vi "SpectralMeasurement_XMutation.vi"(0 "Diagram":refnum<vi>, 5 "ObjRef":refnum<vi>, 6 "Kind":string="SubVI", 7 "Information":string="<Not A Path>") -> (3 "Replace?":bool=TRUE)   [LabVIEW 2020]
uses:
  <vilib>/XNodeSupport/XNodeVersion.ctl
  <vilib>/XNodeSupport/NI_XNodeSupport.lvlib
  <vilib>/XNodeSupport/XNodeState.ctl
  <vilib>/XNodeSupport/XNodeUShort.ctl
  <vilib>/Utility/traverseref.llb/TRef TravTarget.ctl
  <vilib>/XNodeSupport/XNodeVariant.ctl
  <vilib>/Utility/miscctls.llb/LVPositionTypeDef.ctl
  <vilib>/express/express analysis/Spectral/XNode/ExpressSpectralMeasurementsBlockNode.xnode
  <vilib>/BlockNodeSupport/TerminalData.ctl
  <vilib>/picture/picture.llb/imagedata.ctl
  <vilib>/BlockNodeSupport/BlockNodeState.ctl
  <vilib>/XNodeSupport/XNodeType.ctl
  <vilib>/express/express shared/XNodes/controls/ExpressTerminalInfo.ctl
  <vilib>/express/express shared/XNodes/controls/ExpressState.ctl
  <vilib>/express/express shared/XNodes/controls/ExpressBlockNodeState.ctl
panel:
  in  "ExpressBlockNodeState":T1={"BlockNodeState"={"Terminal Data"=[{"Terminal Name"="Signals", "Terminal Display Name"="Signals", "Terminal ID"="Signals", "Terminal Flags"=517, "Terminal Type"=variant(waveform(dbl) {"t0"=timestamp(0 s since 1904-01-01), "dt"=0.0, "Y"=[]}), "Terminal Map ID"=0}, {"Terminal Name"="Selected Measurements", "Terminal Display Name"="Selected Measurements", "Terminal ID"="Selected Measurements", "Terminal Flags"=769, "Terminal Type"=variant(u32 0), "Terminal Map ID"=1}, {"Terminal Name"="Restart Averaging", "Terminal Display Name"="Restart Averaging", "Terminal ID"="Restart Averaging", "Terminal Flags"=769, "Terminal Type"=variant(bool FALSE), "Terminal Map ID"=2}, {"Terminal Name"="View", "Terminal Display Name"="View", "Terminal ID"="View", "Terminal Flags"=769, "Terminal Type"=variant(cluster{"dB On (F)":bool, "unwrap phase (F)":bool, "convert to degree (F)":bool} {"dB On (F)"=FALSE, "unwrap phase (F)"=FALSE, "convert to degree (F)"=FALSE}), "Terminal Map ID"=3}, {"Terminal Name"="Spectrum Window", "Terminal Display Name"="Spectrum Window", "Terminal ID"="Spectrum Window", "Terminal Flags"=769, "Terminal Type"=variant(u16 0), "Terminal Map ID"=4}, {"Terminal Name"="Spectrum Averaging Parameters", "Terminal Display Name"="Spectrum Averaging Parameters", "Terminal ID"="Spectrum Averaging Parameters", "Terminal Flags"=769, "Terminal Type"=variant(cluster{"averaging mode":u16, "weighting mode":u16, "number of averages":u32} {"averaging mode"=0, "weighting mode"=0, "number of averages"=0}), "Terminal Map ID"=5}, {"Terminal Name"="All Spectra", "Terminal Display Name"="All Spectra", "Terminal ID"="All Spectra", "Terminal Flags"=769, "Terminal Type"=variant(bool FALSE), "Terminal Map ID"=6}, {"Terminal Name"="error in (no error)", "Terminal Display Name"="error in (no error)", "Terminal ID"="error in (no error)", "Terminal Flags"=513, "Terminal Type"=variant(errorcluster {"status"=FALSE, "code"=0, "source"=""}), "Terminal Map ID"=7}, {"Terminal Name"="Measurement Output", "Terminal Display Name"="Measurement Output", "Terminal ID"="Measurement Output", "Terminal Flags"=525, "Terminal Type"=variant(dynamicdata []), "Terminal Map ID"=8}, {"Terminal Name"="averaging done", "Terminal Display Name"="averaging done", "Terminal ID"="averaging done", "Terminal Flags"=777, "Terminal Type"=variant(bool FALSE), "Terminal Map ID"=9}, {"Terminal Name"="Phase", "Terminal Display Name"="Phase", "Terminal ID"="Phase", "Terminal Flags"=777, "Terminal Type"=variant(dynamicdata []), "Terminal Map ID"=10}, {"Terminal Name"="error out", "Terminal Display Name"="error out", "Terminal ID"="error out", "Terminal Flags"=521, "Terminal Type"=variant(errorcluster {"status"=FALSE, "code"=0, "source"=""}), "Terminal Map ID"=11}], "Instance Name"="Spectral Measurements", "Type Name"="Spectral Measurements", "Draw Style"=1, "Connector Pane Pattern"=4833, "Flags"=370, "Grown Terminal List Order"=[], "Image"={"image type"=0, "image depth"=8, "image"=[0, 0, 255, 255, 255, 255, 255, 255, 255, 255, 255, 255, 255, 255, 255, 255, 255, 255, 255, 255, 255, 255, 255, 255, 255, 255, 255, 255, 255, 255, 0, 0, 0, 255, 210, 210, 210, 210, 210, 210, 210, 210, 210, 210, 210, 210, 210, 210, 210, 210, 210, 210, 210, 210, 210, 210, 210, 210, 210, 210, 210, 210, 255, 0, 255, 210, 210, 210, 210, 210, 210, 210, 210, 210, 210, 210, 210, 210, 210, 210, 210, 210, 210, 210, 210, 210, 210, 210, 210, 210, 210, 210, 210, 210, 210, 255, 255, 0, 0, 0, 0, 0, 0, 0, 0, 0, 0, 0, 0, 0, 0, 0, 0, 0, 0, 0, 0, 0, 0, 0, 0, 0, 0, 0, 0, 0, 0, 255, 255, 0, 0, 0, 0, 0, 0, 0, 0, 0, 0, 0, 0, 0, 0, 0, 0, 0, 0, 0, 0, 0, 0, 0, 0, 0, 0, 0, 0, 0, 0, 255, 255, 0, 0, 0, 0, 0, 0, 0, 0, 0, 0, 0, 0, 0, 0, 86, 86, 86, 86, 86, 86, 86, 86, 86, 86, 86, 86, 86, 86, 86, 86, 255, 255, 0, 0, 0, 0, 0, 0, 0, 0, 0, 0, 0, 0, 0, 0, 255, 255, 255, 255, 255, 255, 255, 255, 255, 255, 255, 255, 255, 255, 255, 255, 255, 255, 0, 0, 250, 250, 0, 0, 0, 0, 0, 0, 0, 0, 0, 0, 255, 5, 5, 5, 5, 5, 5, 5, 5, 5, 5, 5, 5, 5, 5, 5, 255, 255, 0, 0, 0, 250, 0, 0, 0, 0, 0, 0, 0, 0, 0, 0, 255, 5, 255, 5, 5, 5, 255, 5, 5, 5, 255, 5, 5, 5, 255, 5, 255, 255, 0, 0, 0, 250, 0, 0, 0, 0, 0, 0, 0, 0, 0, 0, 255, 5, 255, 5, 255, 5, 255, 5, 255, 5, 255, 5, 255, 5, 255, 5, 255, 255, 0, 0, 0, 250, 0, 0, 0, 0, 0, 0, 0, 0, 0, 0, 255, 255, 255, 255, 255, 255, 255, 255, 255, 255, 255, 255, 255, 255, 255, 255, 255, 255, 0, 0, 250, 250, 0, 0, 0, 0, 0, 0, 0, 0, 0, 0, 0, 0, 0, 0, 0, 0, 0, 0, 0, 0, 0, 0, 0, 0, 0, 0, 255, 255, 0, 0, 0, 250, 0, 0, 0, 0, 0, 0, 0, 0, 0, 0, 0, 0, 0, 0, 0, 0, 0, 0, 0, 0, 0, 0, 0, 0, 0, 0, 255, 255, 0, 0, 0, 250, 0, 0, 0, 0, 0, 0, 0, 0, 0, 0, 0, 0, 0, 0, 0, 0, 0, 0, 0, 0, 0, 0, 0, 0, 0, 0, 255, 255, 0, 0, 0, 250, 0, 0, 0, 0, 255, 0, 0, 0, 0, 0, 0, 0, 0, 0, 0, 0, 0, 0, 0, 0, 0, 0, 0, 0, 0, 0, 255, 255, 0, 0, 250, 250, 0, 0, 0, 0, 255, 0, 0, 0, 0, 0, 0, 0, 0, 0, 0, 0, 0, 0, 0, 0, 0, 0, 0, 0, 0, 0, 255, 255, 0, 0, 0, 250, 0, 0, 0, 0, 255, 0, 0, 0, 0, 0, 0, 0, 0, 0, 0, 0, 0, 0, 0, 0, 0, 0, 0, 0, 0, 0, 255, 255, 0, 0, 0, 250, 0, 0, 0, 0, 255, 0, 0, 0, 0, 0, 0, 0, 0, 0, 0, 0, 0, 0, 0, 0, 0, 0, 0, 0, 0, 0, 255, 255, 0, 0, 0, 250, 0, 0, 0, 0, 255, 0, 0, 0, 0, 0, 0, 0, 0, 0, 0, 0, 0, 0, 0, 0, 0, 0, 0, 0, 0, 0, 255, 255, 0, 0, 250, 250, 0, 0, 0, 0, 255, 0, 0, 0, 0, 0, 0, 0, 0, 0, 0, 0, 0, 0, 0, 0, 0, 0, 0, 0, 0, 0, 255, 255, 0, 0, 0, 250, 0, 0, 0, 255, 255, 255, 0, 0, 0, 0, 0, 0, 0, 0, 0, 0, 0, 0, 0, 0, 0, 0, 0, 0, 0, 0, 255, 255, 0, 0, 0, 250, 0, 0, 0, 255, 255, 255, 0, 0, 0, 0, 0, 0, 0, 0, 0, 0, 0, 0, 0, 0, 0, 0, 0, 0, 0, 0, 255, 255, 0, 0, 0, 250, 0, 0, 0, 255, 255, 255, 255, 0, 0, 0, 0, 0, 0, 0, 0, 0, 0, 0, 0, 0, 0, 0, 0, 0, 0, 0, 255, 255, 0, 0, 250, 250, 0, 0, 255, 255, 0, 0, 255, 0, 0, 0, 0, 0, 0, 0, 0, 0, 0, 0, 0, 0, 0, 0, 0, 0, 0, 0, 255, 255, 0, 0, 0, 250, 255, 255, 255, 255, 0, 0, 255, 255, 0, 0, 0, 0, 0, 0, 0, 0, 0, 0, 0, 0, 0, 0, 0, 0, 0, 0, 255, 255, 0, 0, 0, 250, 0, 255, 0, 0, 0, 0, 0, 255, 255, 255, 255, 255, 255, 255, 255, 255, 255, 255, 255, 255, 255, 255, 0, 0, 0, 0, 255, 255, 0, 0, 0, 250, 0, 0, 0, 0, 0, 0, 0, 0, 0, 0, 0, 0, 0, 0, 0, 0, 0, 0, 0, 0, 0, 0, 0, 0, 0, 0, 255, 255, 0, 0, 250, 250, 250, 250, 250, 250, 250, 250, 250, 250, 250, 250, 250, 250, 250, 250, 250, 250, 250, 250, 250, 250, 250, 250, 250, 250, 0, 0, 255, 255, 0, 0, 0, 250, 0, 0, 0, 250, 0, 0, 0, 250, 0, 0, 0, 250, 0, 0, 0, 250, 0, 0, 0, 250, 0, 0, 0, 250, 0, 0, 255, 255, 0, 0, 0, 0, 0, 0, 0, 0, 0, 0, 0, 0, 0, 0, 0, 0, 0, 0, 0, 0, 0, 0, 0, 0, 0, 0, 0, 0, 0, 0, 255, 0, 255, 0, 0, 0, 0, 0, 0, 0, 0, 0, 0, 0, 0, 0, 0, 0, 0, 0, 0, 0, 0, 0, 0, 0, 0, 0, 0, 0, 0, 255, 0, 0, 0, 255, 255, 255, 255, 255, 255, 255, 255, 255, 255, 255, 255, 255, 255, 255, 255, 255, 255, 255, 255, 255, 255, 255, 255, 255, 255, 255, 255, 0, 0], "mask"=[63, 255, 255, 252, 127, 255, 255, 254, 255, 255, 255, 255, 255, 255, 255, 255, 255, 255, 255, 255, 255, 255, 255, 255, 255, 255, 255, 255, 255, 255, 255, 255, 255, 255, 255, 255, 255, 255, 255, 255, 255, 255, 255, 255, 255, 255, 255, 255, 255, 255, 255, 255, 255, 255, 255, 255, 255, 255, 255, 255, 255, 255, 255, 255, 255, 255, 255, 255, 255, 255, 255, 255, 255, 255, 255, 255, 255, 255, 255, 255, 255, 255, 255, 255, 255, 255, 255, 255, 255, 255, 255, 255, 255, 255, 255, 255, 255, 255, 255, 255, 255, 255, 255, 255, 255, 255, 255, 255, 255, 255, 255, 255, 255, 255, 255, 255, 255, 255, 255, 255, 127, 255, 255, 254, 63, 255, 255, 252], "colors"=[16777215, 16777164, 16777113, 16777062, 16777011, 16776960, 16764159, 16764108, 16764057, 16764006, 16763955, 16763904, 16751103, 16751052, 16751001, 16750950, 16750899, 16750848, 16738047, 16737996, 16737945, 16737894, 16737843, 16737792, 16724991, 16724940, 16724889, 16724838, 16724787, 16724736, 16711935, 16711884, 16711833, 16711782, 16711731, 16711680, 13434879, 13434828, 13434777, 13434726, 13434675, 13434624, 13421823, 13421772, 13421721, 13421670, 13421619, 13421568, 13408767, 13408716, 13408665, 13408614, 13408563, 13408512, 13395711, 13395660, 13395609, 13395558, 13395507, 13395456, 13382655, 13382604, 13382553, 13382502, 13382451, 13382400, 13369599, 13369548, 13369497, 13369446, 13369395, 13369344, 10092543, 10092492, 10092441, 10092390, 10092339, 10092288, 10079487, 10079436, 10079385, 10079334, 10079283, 10079232, 10066431, 10066380, 10066329, 10066278, 10066227, 10066176, 10053375, 10053324, 10053273, 10053222, 10053171, 10053120, 10040319, 10040268, 10040217, 10040166, 10040115, 10040064, 10027263, 10027212, 10027161, 10027110, 10027059, 10027008, 6750207, 6750156, 6750105, 6750054, 6750003, 6749952, 6737151, 6737100, 6737049, 6736998, 6736947, 6736896, 6724095, 6724044, 6723993, 6723942, 6723891, 6723840, 6711039, 6710988, 6710937, 6710886, 6710835, 6710784, 6697983, 6697932, 6697881, 6697830, 6697779, 6697728, 6684927, 6684876, 6684825, 6684774, 6684723, 6684672, 3407871, 3407820, 3407769, 3407718, 3407667, 3407616, 3394815, 3394764, 3394713, 3394662, 3394611, 3394560, 3381759, 3381708, 3381657, 3381606, 3381555, 3381504, 3368703, 3368652, 3368601, 3368550, 3368499, 3368448, 3355647, 3355596, 3355545, 3355494, 3355443, 3355392, 3342591, 3342540, 3342489, 3342438, 3342387, 3342336, 65535, 65484, 65433, 65382, 65331, 65280, 52479, 52428, 52377, 52326, 52275, 52224, 39423, 39372, 39321, 39270, 39219, 39168, 26367, 26316, 26265, 26214, 26163, 26112, 13311, 13260, 13209, 13158, 13107, 13056, 255, 204, 153, 102, 51, 15597568, 14483456, 12255232, 11141120, 8912896, 7798784, 5570560, 4456448, 2228224, 1114112, 60928, 56576, 47872, 43520, 34816, 30464, 21760, 17408, 8704, 4352, 238, 221, 187, 170, 136, 119, 85, 68, 34, 17, 15658734, 14540253, 12303291, 11184810, 8947848, 7829367, 5592405, 4473924, 2236962, 1118481, 0], "Rectangle"={"left"=0, "top"=0, "right"=32, "bottom"=32}}}, "ExpressState"={"Terminal Info"=[{"types to adapt"=["ExpressData", "Waveform", "1D Array Waveform"], "show config value"=FALSE, "default type"=variant(waveform(dbl) {"t0"=timestamp(0 s since 1904-01-01), "dt"=0.0, "Y"=[]}), "display name control"=""}, {"types to adapt"=["Numeric"], "show config value"=FALSE, "default type"=variant(u32 0), "display name control"=""}, {"types to adapt"=["Boolean"], "show config value"=FALSE, "default type"=variant(bool FALSE), "display name control"=""}, {"types to adapt"=[""], "show config value"=FALSE, "default type"=variant(cluster{"dB On (F)":bool, "unwrap phase (F)":bool, "convert to degree (F)":bool} {"dB On (F)"=FALSE, "unwrap phase (F)"=FALSE, "convert to degree (F)"=FALSE}), "display name control"=""}, {"types to adapt"=["Numeric"], "show config value"=FALSE, "default type"=variant(u16 0), "display name control"=""}, {"types to adapt"=[""], "show config value"=FALSE, "default type"=variant(cluster{"averaging mode":u16, "weighting mode":u16, "number of averages":u32} {"averaging mode"=0, "weighting mode"=0, "number of averages"=0}), "display name control"=""}, {"types to adapt"=["Boolean"], "show config value"=FALSE, "default type"=variant(bool FALSE), "display name control"=""}, {"types to adapt"=[""], "show config value"=FALSE, "default type"=variant(errorcluster {"status"=FALSE, "code"=0, "source"=""}), "display name control"=""}, {"types to adapt"=["ExpressData"], "show config value"=FALSE, "default type"=variant(dynamicdata []), "display name control"="output name"}, {"types to adapt"=["Boolean"], "show config value"=FALSE, "default type"=variant(bool FALSE), "display name control"=""}, {"types to adapt"=["ExpressData"], "show config value"=FALSE, "default type"=variant(dynamicdata []), "display name control"=""}, {"types to adapt"=[""], "show config value"=FALSE, "default type"=variant(errorcluster {"status"=FALSE, "code"=0, "source"=""}), "display name control"=""}], "config control names"=[], "config data strings"=[], "config control data"=[variant(enum32{"Magnitude (RMS)", "Magnitude (Peak)", "Power spectrum", "Power spectral density"} enum."Magnitude (RMS)"), variant(enum32{"Linear", "dB"} enum."dB"), variant(u16 0), variant(bool FALSE), variant(enum32{"Vector", "RMS", "Peak hold"} enum."Vector"), variant(enum32{"Linear", "Exponential"} enum."Linear"), variant(u32 1), variant(enum32{"Every iteration", "Only when averaging complete"} enum."Every iteration"), variant(bool FALSE), variant(bool FALSE), variant(bool FALSE), variant(waveform(dbl)[] []), variant(waveform(dbl) {"t0"=timestamp(0 s since 1904-01-01), "dt"=1.0, "Y"=[]}), variant(errorcluster {"status"=FALSE, "code"=0, "source"=""}), variant(dynamicdata []), variant(cluster{"dB On (F)":bool, "unwrap phase (F)":bool, "convert to degree (F)":bool} {"dB On (F)"=FALSE, "unwrap phase (F)"=FALSE, "convert to degree (F)"=FALSE}), variant(cluster{"averaging mode":enum16{"No averaging", "Vector averaging", "RMS averaging", "Peak hold"}, "weighting mode":enum16{"Linear", "Exponential"}, "number of averages":u32} {"averaging mode"=enum."No averaging", "weighting mode"=enum."Linear", "number of averages"=0}), variant(string "Sample Data"), variant(string "Sample Result"), variant(waveform(dbl) {"t0"=timestamp(0 s since 1904-01-01), "dt"=1.0, "Y"=[]}), variant(string "Sample Result"), variant(string "Phase (rad.)"), variant(string "Phase (deg.)"), variant(bool FALSE), variant(bool FALSE), variant(string[] ["INsignal type", "INfrequency", "OUTsignal", "INphase", "INsamples per second"]), variant(string[] ["INsignal type", "INfrequency", "OUTsignal"]), variant(errorcluster {"status"=FALSE, "code"=0, "source"=""}), variant(bool FALSE), variant(dynamicdata []), variant(string[] ["FFT - (RMS)", "FFT - (Peak)", "Power Spectrum", "PSD"]), variant(string ""), variant(bool FALSE), variant(bool FALSE), variant(i32 0), variant(string ""), variant(bool FALSE), variant(bool FALSE), variant(bool FALSE), variant(enum16{"No averaging", "Vector averaging", "RMS averaging", "Peak hold"} enum."No averaging"), variant(enum16{"Linear", "Exponential"} enum."Linear"), variant(u32 0), variant(bool FALSE), variant(i32 0), variant(string "")], "units"=[], "configured?"=TRUE, "config VI path"=path "<vilib>/express/express analysis/Spectral/Config/ExnSpectralConfig Configure Spectral Measurements.vi", "block VI path"=path "<vilib>/express/express analysis/Spectral/Block/ExnSpectralBlock Spectral Measurements.vi", "config control labels"=["Selected Measurement", "Result", "Spectrum Window", "Averaging", "Mode", "Weighting", "Number of averages", "Produce Spectrum", "Unwrap phase", "Convert to degree", "Correction None", " Windowed Signal ", "Magnitude", "error out", "Signals", "View", "Spectrum Averaging Parameters", "Sample Input Signal", "Sample Magnitude Result", "Phase", "Sample Phase Result", "Phase (rad.)", "Phase (deg.)", "Restart Averaging", "okay out", "config terms", "config terms grown", "error in (no error)", "averaging done", "Measurement Output", "measurement names", "output name", "All Spectra", "status", "code", "source", "dB On (F)", "unwrap phase (F)", "convert to degree (F)", "averaging mode", "weighting mode", "number of averages", "status", "code", "source"], "show config value menu"=FALSE, "config value menu setting"=FALSE, "context help labels"=["Selected Measurement", "Result", "Spectrum Window", "Averaging", "Mode", "Weighting", "Number of averages", "Produce Spectrum", "Unwrap phase", "Convert to degree"], "valid help labels"=[]}} {"BlockNodeState"."Draw Style" items=["FunctionBlock", "ExpressVI", "Variable", "Elemental I/O", "32x32 Icon", "FunctionBlockCompact"]; "BlockNodeState"."Terminal Data"."Terminal Flags" format="%.0b"}
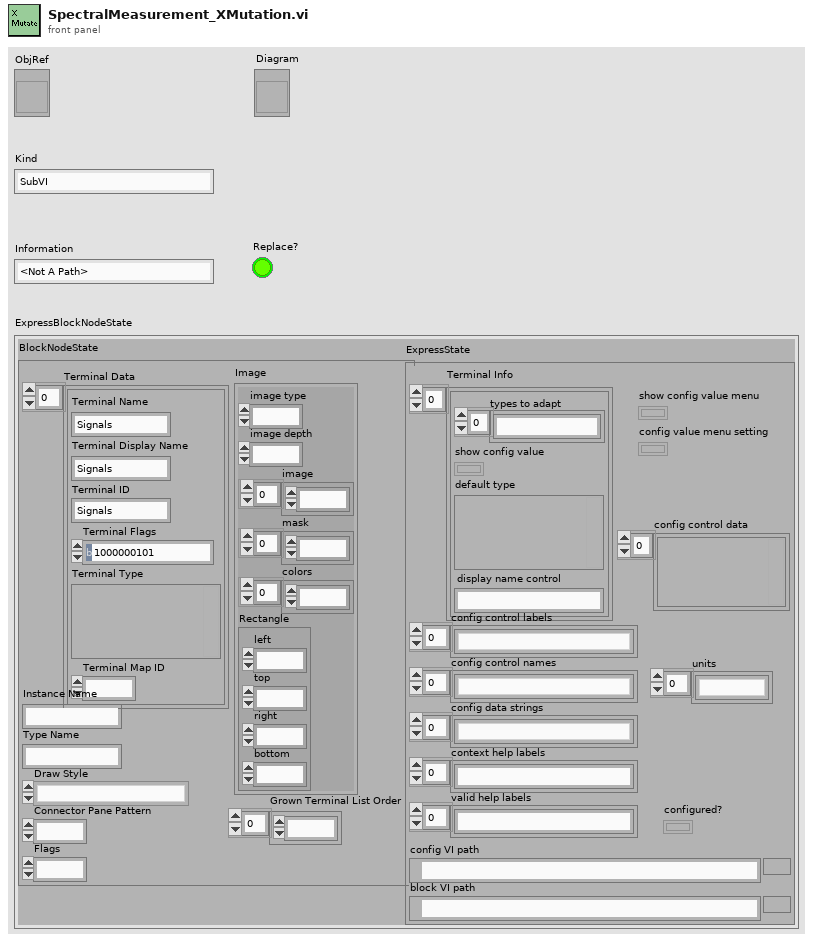
[diagram p1: front panel]
types:
  T1 = typedef "ExpressBlockNodeState.ctl" = cluster{"BlockNodeState":T2, "ExpressState":T5}
  T2 = typedef "BlockNodeState.ctl" = cluster{"Terminal Data":T3[], "Instance Name":string, "Type Name":string, "Draw Style":i32, "Connector Pane Pattern":i32, "Flags":i32, "Grown Terminal List Order":i32[], "Image":T4}
  T3 = typedef "TerminalData.ctl" = cluster{"Terminal Name":string, "Terminal Display Name":string, "Terminal ID":string, "Terminal Flags":i32, "Terminal Type":variant, "Terminal Map ID":i32}
  T4 = typedef "imagedata.ctl" = cluster{"image type":i32, "image depth":i32, "image":u8[], "mask":u8[], "colors":u32[], "Rectangle":cluster{"left":i16, "top":i16, "right":i16, "bottom":i16}}
  T5 = typedef "ExpressState.ctl" = cluster{"Terminal Info":T6, "config control names":string[], "config data strings":string[], "config control data":variant[], "units":string[], "configured?":bool, "config VI path":path, "block VI path":path, "config control labels":string[], "show config value menu":bool, "config value menu setting":bool, "context help labels":string[], "valid help labels":string[]}
  T6 = typedef "ExpressTerminalInfo.ctl" = cluster{"types to adapt":string[], "show config value":bool, "default type":T7, "display name control":string}[]
  T7 = typedef "NI_XNodeSupport.lvlib/XNodeType.ctl" = variant
  T8 = cluster{"dB On (F)":bool, "unwrap phase (F)":bool, "convert to degree (F)":bool}
  T9 = cluster{"averaging mode":enum16{"No averaging", "Vector averaging", "RMS averaging", "Peak hold"}, "weighting mode":enum16{"Linear", "Exponential"}, "number of averages":u32}
  T10 = typedef "TRef TravTarget.ctl" = enum16{"FP", "BD", "Other"}
  T11 = enum32{"Every iteration", "Only when averaging complete"}
  T12 = enum32{"Magnitude (RMS)", "Magnitude (Peak)", "Power spectrum", "Power spectral density"}
  T13 = typedef "NI_XNodeSupport.lvlib/XNodeState.ctl" = cluster{"Version":T14, "State Data":T16}
  T14 = typedef "NI_XNodeSupport.lvlib/XNodeVersion.ctl" = cluster{"Major":T15, "Minor":T15, "Fix":T15, "Build":T15}
  T15 = typedef "NI_XNodeSupport.lvlib/XNodeUShort.ctl" = u16
  T16 = typedef "NI_XNodeSupport.lvlib/XNodeVariant.ctl" = variant
  T17 = typedef "LVPositionTypeDef.ctl" = cluster{"Left":i32, "Top":i32}
  T18 = enum16{"No averaging", "Vector averaging", "RMS averaging", "Peak hold"}
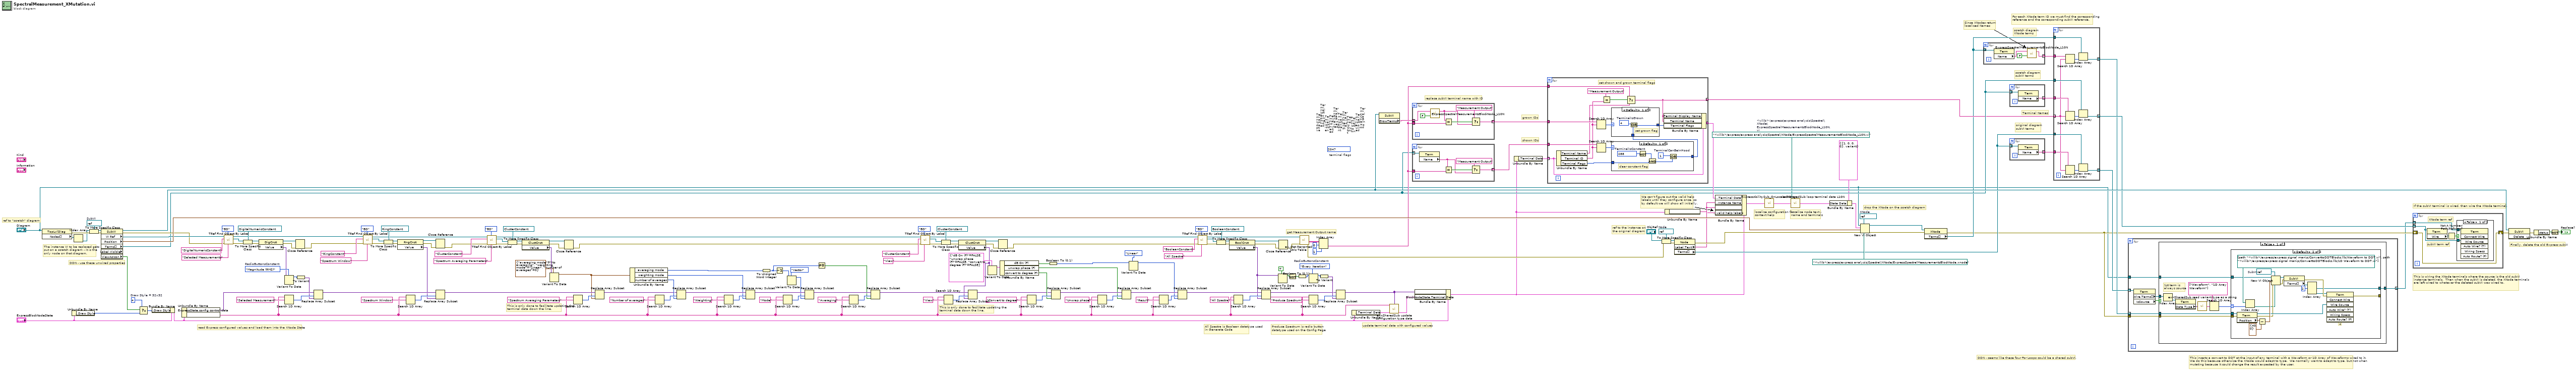
[diagram p0: block diagram]
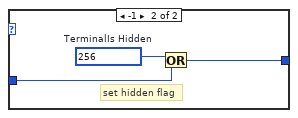
[diagram p4: hidden frame]
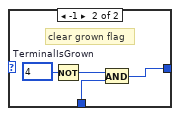
[diagram p5: hidden frame]
diagram:
  w3 = path "<vilib>/express/express analysis/Spectral/XNode/ExpressSpectralMeasurementsBlockNode_L10N.vi"  # <vilib>:\express\express analysis\Spectral\XNode\ExpressSpectralMeasurementsBlockNode_L10N.vi
  w21 = 4  # Draw Style = 32x32
  (unwired) 2047 ("TermFlags")
  w105 = T11."Every iteration"  # RadioButtonsConstant
  w65 = T12."Magnitude (RMS)"  # RadioButtonsConstant
  w184 = refnum<vi> refnum  # Node
  w191 = refnum<vi> refnum  # XNode
  w196 = refnum<vi> refnum  # SubVI
  # "Since XNodes return localized Names"
  # "We can't figure out the valid help labels until they configure once, so by default we will show all initially."
  # "localize node text - name and terminals"
  # "localize configuration for context help"
  # "scratch diagram\nXNode terms"
  # "scratch diagram\nsubVI terms"
  # "This inserts a convert to DDT at the input of any terminal with a Waveform or 1D Array of Waveforms wired to it.  We do this because otherwise the XNode would adapt to type.  We normally want to adapt to type, but not when mutating because it could change the result expected by the user."
  # "original diagram\nsubVI terms"
  # "Produce Spectrum is radio button datatype used on the Config Page"
  # "All Spectra is Boolean datatype used in Generate Code"
  # "DDN - seems like these four For Loops could be a shared subVI."
  # "DDN - use these unwired properties"
  # "This is only done to facilitate updating the terminal data down the line."
  # "TerminalIsAdaptive"
  # "TerminalIsRecommended"
  # "TerminalIsHidden"
  # "terminal flags"
  # "TerminalIsInverted"
  # "TerminalCanBeInverted"
  # "TerminalIsConstant"
  # "TerminalHilitedMask"
  # "TerminalIsOutput"
  # "TerminalIsGrown"
  # "TerminalIsRequired"
  # "TerminalCanBeInHood"
  # "This is only done to facilitate updating the terminal data down the line."
  # "update terminal data with configured values"
  # "Finally, delete the old Express subVI"
  # "For each XNode term ID we must find the corresponding reference and the corresponding subVI reference."
  # "drop the XNode on the scratch diagram"
  # "read Express configured values and load them into the XNode State"
  # "Terminal Names"
  # "If the subVI terminal is wired, then wire the XNode terminal."
  # "This is wiring the XNode terminals where the source is the old subVI instance terminals.  Then when the subVI is deleted, the XNode terminals are left wired to whatever the deleted subVI was wired to."
  # "The instance VI to be replaced gets put on a scratch diagram - it is the only node on that diagram."
  # "replace subVI terminal name with ID"
  # "grown IDs"
  # "shown IDs"
  # "get Measurement Output name"
  # "ref to \"scratch\" diagram"
  # "ref to the instance on the original diagram"
  n1 = property class="TopLvlDiag"(reference="Diagram") -> (error out=w195:errorcluster, "Nodes[]"=w197:refnum<vi>[])  [unwired: 1 in, 1 out]
  n2 = Unbundle By Name("ExpressBlockNodeState") -> ("BlockNodeState.Draw Style"=w20:i32)
  n3 = Index Array(array=w197) -> (element=w187:refnum<vi>)  [unwired: 1 in]
  n4 = To More Specific Class(target class=w196, reference=w187, error in=w195) -> (specific class reference=w193:refnum<vi>, error out=w194:errorcluster)
  n5 = property class="SubVI" props=["VI Ref", "Position", "Terms[]", "Label", "Visible", "ViewAsIcon"](reference=w193, error in=w194) -> (reference out=w91:refnum<vi>, error out=w172:errorcluster, "VI Ref"=w173:refnum<vi>, "Position"=w174:T17, "Terms[]"=w90:refnum<vi>[], "ViewAsIcon"=w22:bool)  [unwired: 1 out]
  n6 = Select(t=w21, s=w22, f=w20) -> (s? t:f=w23:i32)
  n7 = Bundle By Name(cluster="ExpressBlockNodeState", "BlockNodeState.Draw Style"=w23) -> (w24:T1)
  n8 = Unbundle By Name(w24) -> ("ExpressState.config control data"=w170:variant[], "ExpressState.config control labels"=w14:string[])
  n9 = call <vilib>:"TRef Find Object By Label.vi"("Label"="Selected Measurements", "Traverse Target"=TRef_TravTarget."BD", "error in (no error)"=w172, "Class Name"="DigitalNumericConstant" ("Label"), "VI Ref"=w173) -> ("error out"=w180:errorcluster, "Found Obj Ref"=w178:refnum<vi>, "dup VI Ref"=w157:refnum<vi>)  [unwired: 3 in, 1 out]
  n10 = To More Specific Class(target class=refnum<vi> refnum ("Other Refnum"), reference=w178, error in=w180) -> (specific class reference=w176:refnum<vi>, error out=w177:errorcluster)
  n11 = property class="DigCnst"(reference=w176, error in=w177) -> (reference out=w168:refnum<vi>, error out=w167:errorcluster, "Value"=w63:variant)
  n12 = Variant To Data(type=w65, Variant=w63) -> (data=w64:T12)  [unwired: 1 in, 1 out]
  n13 = Search 1D Array(1D array=w14, element="Selected Measurement" ("Label")) -> (index of element=w169:i32)  [unwired: 1 in]
  n14 = Close Reference(reference=w168, error in (no error)=w167) -> (error out=w156:errorcluster)
  n15 = To Variant(anything=w64) -> (Variant=w62:variant)
  n16 = Replace Array Subset(array=w170, new element=w62, index=w169) -> (w154:variant[])
  n17 = call <vilib>:"TRef Find Object By Label.vi"("Label"="Spectrum Window", "Traverse Target"=TRef_TravTarget."BD", "error in (no error)"=w156, "Class Name"="RingConstant" ("Label"), "VI Ref"=w157) -> ("error out"=w163:errorcluster, "Found Obj Ref"=w162:refnum<vi>, "dup VI Ref"=w141:refnum<vi>)  [unwired: 3 in, 1 out]
  n18 = To More Specific Class(target class=refnum<vi> refnum ("Other Refnum"), reference=w162, error in=w163) -> (specific class reference=w160:refnum<vi>, error out=w161:errorcluster)
  n19 = property class="RngCnst"(reference=w160, error in=w161) -> (reference out=w159:refnum<vi>, error out=w158:errorcluster, "Value"=w152:variant)
  n20 = Search 1D Array(1D array=w14, element="Spectrum Window" ("Label")) -> (index of element=w153:i32)  [unwired: 1 in]
  n21 = Close Reference(reference=w159, error in (no error)=w158) -> (error out=w140:errorcluster)
  n22 = Replace Array Subset(array=w154, new element=w152, index=w153) -> (w33:variant[])
  n23 = call <vilib>:"TRef Find Object By Label.vi"("Label"="Spectrum Averaging Parameters", "Traverse Target"=TRef_TravTarget."BD", "error in (no error)"=w140, "Class Name"="ClusterConstant" ("Label"), "VI Ref"=w141) -> ("error out"=w148:errorcluster, "Found Obj Ref"=w149:refnum<vi>, "dup VI Ref"=w83:refnum<vi>)  [unwired: 3 in, 1 out]
  n24 = To More Specific Class(target class=refnum<vi> refnum ("Other Refnum"), reference=w149, error in=w148) -> (specific class reference=w151:refnum<vi>, error out=w150:errorcluster)
  n25 = property class="ClustCnst"(reference=w151, error in=w150) -> (reference out=w143:refnum<vi>, error out=w142:errorcluster, "Value"=w81:variant)
  n26 = Variant To Data(type=T9 {"averaging mode"=enum."No averaging", "weighting mode"=enum."Linear", "number of averages"=0} ("Spectrum Averaging Parameters"), Variant=w81) -> (data=w31:T9)  [unwired: 1 in, 1 out]
  n27 = Close Reference(reference=w143, error in (no error)=w142) -> (error out=w126:errorcluster)
  n28 = Search 1D Array(1D array=w14, element="Spectrum Averaging Parameters" ("Label")) -> (index of element=w34:i32)  [unwired: 1 in]
  n29 = Replace Array Subset(array=w33, new element=w31, index=w34) -> (w32:variant[])
  n30 = Unbundle By Name(w31) -> ("averaging mode"=w67:T18, "weighting mode"=w69:enum16{"Linear", "Exponential"}, "number of averages"=w79:u32)
  n31 = Search 1D Array(1D array=w14, element="Number of averages" ("Label")) -> (index of element=w139:i32)  [unwired: 1 in]
  n32 = Replace Array Subset(array=w32, new element=w79, index=w139) -> (w76:variant[])
  n33 = Search 1D Array(1D array=w14, element="Weighting" ("Label")) -> (index of element=w77:i32)  [unwired: 1 in]
  n34 = Replace Array Subset(array=w76, new element=w69, index=w77) -> (w73:variant[])
  n35 = To Unsigned Word Integer(number=w67) -> (unsigned 16bit integer=w66:u16)
  n36 = Decrement(x=w66) -> (x-1=w61:u16)
  n37 = Search 1D Array(1D array=w14, element="Mode" ("Label")) -> (index of element=w75:i32)  [unwired: 1 in]
  n38 = Variant To Data(type=enum32{"Vector", "RMS", "Peak hold"}."Vector" ("Mode"), Variant=w61) -> (data=w60:enum32{"Vector", "RMS", "Peak hold"})  [unwired: 1 in, 1 out]
  n39 = Replace Array Subset(array=w73, new element=w60, index=w75) -> (w70:variant[])
  n40 = Not Equal To 0?(x=w66) -> (x != 0?=w68:bool)
  n41 = Search 1D Array(1D array=w14, element="Averaging" ("Label")) -> (index of element=w71:i32)  [unwired: 1 in]
  n42 = Replace Array Subset(array=w70, new element=w68, index=w71) -> (w28:variant[])
  n43 = call <vilib>:"TRef Find Object By Label.vi"("Label"="View", "Traverse Target"=TRef_TravTarget."BD", "error in (no error)"=w126, "Class Name"="ClusterConstant" ("Label"), "VI Ref"=w83) -> ("error out"=w132:errorcluster, "Found Obj Ref"=w131:refnum<vi>, "dup VI Ref"=w112:refnum<vi>)  [unwired: 3 in, 1 out]
  n44 = To More Specific Class(target class=refnum<vi> refnum ("Other Refnum"), reference=w131, error in=w132) -> (specific class reference=w129:refnum<vi>, error out=w130:errorcluster)
  n45 = Search 1D Array(1D array=w14, element="View" ("Label")) -> (index of element=w30:i32)  [unwired: 1 in]
  n46 = property class="ClustCnst"(reference=w129, error in=w130) -> (reference out=w128:refnum<vi>, error out=w127:errorcluster, "Value"=w26:variant)
  n47 = Replace Array Subset(array=w28, new element=w26, index=w30) -> (w27:variant[])
  n48 = Variant To Data(type=T8 {"dB On (F)"=FALSE, "unwrap phase (F)"=FALSE, "convert to degree (F)"=FALSE} ("View"), Variant=w26) -> (data=w57:T8)  [unwired: 1 in, 1 out]
  n49 = Close Reference(reference=w128, error in (no error)=w127) -> (error out=w113:errorcluster)
  n50 = Unbundle By Name(w57) -> ("dB On (F)"=w51:bool, "unwrap phase (F)"=w52:bool, "convert to degree (F)"=w56:bool)
  n51 = Search 1D Array(1D array=w14, element="Convert to degree" ("Label")) -> (index of element=w124:i32)  [unwired: 1 in]
  n52 = Boolean To (0,1)(Boolean=w51) -> (0, 1=w47:i16)
  n53 = Replace Array Subset(array=w27, new element=w56, index=w124) -> (w53:variant[])
  n54 = Search 1D Array(1D array=w14, element="Unwrap phase" ("Label")) -> (index of element=w55:i32)  [unwired: 1 in]
  n55 = Replace Array Subset(array=w53, new element=w52, index=w55) -> (w48:variant[])
  n56 = Variant To Data(type=enum32{"Linear", "dB"}."Linear" ("Result"), Variant=w47) -> (data=w45:enum32{"Linear", "dB"})  [unwired: 1 in, 1 out]
  n57 = Search 1D Array(1D array=w14, element="Result" ("Label")) -> (index of element=w49:i32)  [unwired: 1 in]
  n58 = Replace Array Subset(array=w48, new element=w45, index=w49) -> (w17:variant[])
  n59 = call <vilib>:"TRef Find Object By Label.vi"("Label"="All Spectra", "Traverse Target"=TRef_TravTarget."BD", "error in (no error)"=w113, "Class Name"="BooleanConstant" ("Label"), "VI Ref"=w112) -> ("error out"=w118:errorcluster, "Found Obj Ref"=w119:refnum<vi>, "dup VI Ref"=w102:refnum<vi>)  [unwired: 3 in, 1 out]
  n60 = To More Specific Class(target class=refnum<vi> refnum ("Other Refnum"), reference=w119, error in=w118) -> (specific class reference=w121:refnum<vi>, error out=w120:errorcluster)
  n61 = property class="BoolCnst"(reference=w121, error in=w120) -> (reference out=w122:refnum<vi>, error out=w123:errorcluster, "Value"=w15:variant)
  n62 = Search 1D Array(1D array=w14, element="All Spectra" ("Label")) -> (index of element=w18:i32)  [unwired: 1 in]
  n63 = Replace Array Subset(array=w17, new element=w15, index=w18) -> (w16:variant[])
  n64 = Variant To Data(type=TRUE, Variant=w15) -> (data=w107:bool)  [unwired: 1 in, 1 out]
  n65 = Close Reference(reference=w122, error in (no error)=w123) -> (error out=w101:errorcluster)
  n66 = Not(x=w107) -> (.not. x?=w109:bool)
  n67 = Boolean To (0,1)(Boolean=w109) -> (0, 1=w106:i16)
  n68 = call <vilib>:"ex_Get Renamed Ctrls Table.vi"("error in (no error)"=w101, "VI refnum"=w102) -> ("error out"=w43:errorcluster, "Renamed Controls"=w100:string[][])  [unwired: 6 in, 2 out]
  n69 = Variant To Data(type=w105, Variant=w106) -> (data=w104:T11)  [unwired: 1 in, 1 out]
  n70 = Search 1D Array(1D array=w14, element="Produce Spectrum" ("Label")) -> (index of element=w111:i32)  [unwired: 1 in]
  n71 = Index Array(array=w100, index (row)=0, index (col)=1 ("index (row)")) -> (element=w94:string)
  n72 = To Variant(anything=w104) -> (Variant=w103:variant)
  n73 = Replace Array Subset(array=w16, new element=w103, index=w111) -> (w38:variant[])
  n74 = Unbundle By Name(w24) -> ("BlockNodeState.Terminal Data"=w37:T3[])
  n75 = property class="SubVI"(reference=w91) -> ("GrowTerms"=w97:string[])  [unwired: 1 in, 2 out]
  n76 = call <vilib>:"exnSharedSub update configuration type data.vi"("config control labels"=w14, "config control data"=w38, "Terminal Data in"=w37) -> ("Terminal Data out"=w36:T3[])  [unwired: 12 in]
  n77 = for {
    tunnel: w97 -> [w199] mode=indexing
    tunnel: w94 -> [w204]
    tunnel: [w201] -> w95 mode=indexing
    n78 = call <vilib>:"ExpressSpectralMeasurementsBlockNode_L10N.vi"("Localize? (True)"=FALSE, "String In"=w199) -> ("String Out"=w198:string)  [unwired: 1 in]
    n79 = Equal?(x=w198, y=w204) -> (x = y?=w202:bool)
    n80 = Select(t="Measurement Output", s=w202, f=w198) -> (s? t:f=w201:string)
  }
  n81 = for {
    tunnel: w90 -> [w210] mode=indexing
    tunnel: [w208] -> w87 mode=indexing
    tunnel: w94 -> [w205]
    n82 = property class="Term"(reference=w210) -> ("Name"=w206:string)  [unwired: 1 in, 2 out]
    n83 = Equal?(x=w206, y=w205) -> (x = y?=w209:bool)
    n84 = Select(t="Measurement Output", s=w209, f=w206) -> (s? t:f=w208:string)
  }
  n85 = Bundle By Name(cluster=w24, "ExpressState.config control data"=w38, "BlockNodeState.Terminal Data"=w36) -> (w2:T1)
  n86 = Unbundle By Name(w2) -> ("BlockNodeState.Terminal Data"=w96:T3[])
  n87 = for {
    tunnel: w96 -> [w214] mode=indexing
    tunnel: w87 -> [w225]
    tunnel: w95 -> [w224]
    tunnel: w94 -> [w215]
    tunnel: [w212] -> w93 mode=indexing
    tunnel: [w211] -> w88 mode=indexing
    # "set shown and grown terminal flags"
    n88 = Unbundle By Name(w214) -> ("Terminal Name"=w216:string, "Terminal ID"=w219:string, "Terminal Flags"=w221:i32)
    n89 = Search 1D Array(1D array=w224, element=w219) -> (index of element=w222:i32)  [unwired: 1 in]
    n90 = Search 1D Array(1D array=w225, element=w219) -> (index of element=w223:i32)  [unwired: 1 in]
    n91 = Equal?(x="Measurement Output", y=w219) -> (x = y?=w217:bool)
    n92 = case shown="Default" w223 {
      tunnel: w221 -> [w226 w233]
      tunnel: [w230 w232] -> w220
      frame Default {
        w229 = 288  # TerminalIsConstant
        w231 = 1  # TerminalCanBeInHood
        # "clear constant flag"
        n93 = Not(x=w229) -> (.not. x?=w227:i32)
        n94 = And(x=w227, y=w226) -> (x .and. y?=w228:i32)
        n95 = Or(x=w231, y=w228) -> (x .or. y?=w230:i32)
      }
      frame -1 {
        w234 = 256  # TerminalIs Hidden
        # "set hidden flag"
        n96 = Or(x=w234, y=w233) -> (x .or. y?=w232:i32)
      }
    }
    n97 = case shown="Default" w222 {
      tunnel: w220 -> [w236 w241]
      tunnel: [w235 w239] -> w213
      frame Default {
        w237 = 4  # TerminalIsGrown
        # "set grown flag"
        n98 = Or(x=w237, y=w236) -> (x .or. y?=w235:i32)
      }
      frame -1 {
        w240 = 4  # TerminalIsGrown
        # "clear grown flag"
        n99 = Not(x=w240) -> (.not. x?=w238:i32)
        n100 = And(x=w238, y=w241) -> (x .and. y?=w239:i32)
      }
    }
    n101 = Select(t=w215, s=w217, f=w216) -> (s? t:f=w211:string)
    n102 = Bundle By Name(cluster=w214, "Terminal Display Name"=w211, "Terminal Name"=w211, "Terminal Flags"=w213) -> (w212:T3)
  }
  n103 = To More Specific Class(target class=w184, reference="ObjRef", error in=w43) -> (specific class reference=w185:refnum<vi>, error out=w183:errorcluster)
  n104 = Unbundle By Name(w2) -> ("ExpressState.context help labels"=w1:string[])
  n105 = property class="Node"(reference=w185, error in=w183) -> (error out=w42:errorcluster, "Label.Text"=w41:string, "Terms[]"=w12:refnum<vi>[])  [unwired: 1 out]
  n106 = Bundle By Name(cluster=w2, "BlockNodeState.Terminal Data"=w93, "BlockNodeState.Instance Name"=w41, "BlockNodeState.Type Name"=w41, "ExpressState.valid help labels"=w1) -> (w6:T1)
  n107 = call <vilib>:"ExpressAbilitySub_OnLocaleChange.vi"("State In"=w6) -> ("State Out"=w5:T1)  [unwired: 14 in]
  n108 = call <vilib>:"exnSharedSub loop terminal data L10N.vi"("path to L10N subVI"=w3, "ExpressBlockNodeState In"=w5) -> ("ExpressBlockNodeState Out"=w4:T1)  [unwired: 13 in]
  n109 = Bundle By Name(cluster=T13 {"Version"={"Major"=1, "Minor"=0, "Fix"=0, "Build"=0}, "State Data"=variant} ("State"), "State Data"=w4) -> (w190:T13)
  n110 = New VI Object(vi object class=w191, owner refnum="Diagram", style=w190, position/next to=w174, 6:path "<vilib>/express/express analysis/Spectral/XNode/ExpressSpectralMeasurementsBlockNode.xnode", 8:w42) -> (object refnum=w189:refnum<vi>, 0:w44:errorcluster)  [unwired: 2 in]
  n111 = property class="XNode"(reference=w189, error in=w44) -> (error out=w9:errorcluster, "Terms[]"=w86:refnum<vi>[])  [unwired: 1 out]
  n112 = for {
    tunnel: w86 -> [w245] mode=indexing
    tunnel: [w242] -> w85 mode=indexing
    n113 = property class="Term"(reference=w245) -> ("Name"=w243:string)  [unwired: 1 in, 2 out]
    n114 = call <vilib>:"ExpressSpectralMeasurementsBlockNode_L10N.vi"("Localize? (True)"=FALSE, "String In"=w243) -> ("String Out"=w242:string)  [unwired: 1 in]
  }
  n115 = for {
    tunnel: w90 -> [w247] mode=indexing
    tunnel: [w246] -> w89 mode=indexing
    n116 = property class="Term"(reference=w247) -> ("Name"=w246:string)  [unwired: 1 in, 2 out]
  }
  n117 = for {
    tunnel: w12 -> [w249] mode=indexing
    tunnel: [w248] -> w13 mode=indexing
    n118 = property class="Term"(reference=w249) -> ("Name"=w248:string)  [unwired: 1 in, 2 out]
  }
  n119 = for {
    tunnel: w86 -> [w257]
    tunnel: w90 -> [w260]
    tunnel: w89 -> [w261]
    tunnel: w88 -> [w251] mode=indexing
    tunnel: [w259] -> w84 mode=indexing
    tunnel: w85 -> [w256]
    tunnel: [w255] -> w10 mode=indexing
    tunnel: w12 -> [w254]
    tunnel: w13 -> [w253]
    tunnel: [w250] -> w11 mode=indexing
    n120 = Search 1D Array(1D array=w256, element=w251) -> (index of element=w258:i32)  [unwired: 1 in]
    n121 = Search 1D Array(1D array=w261, element=w251) -> (index of element=w262:i32)  [unwired: 1 in]
    n122 = Search 1D Array(1D array=w253, element=w251) -> (index of element=w252:i32)  [unwired: 1 in]
    n123 = Index Array(array=w257, index=w258) -> (element=w255:refnum<vi>)
    n124 = Index Array(array=w260, index=w262) -> (element=w259:refnum<vi>)
    n125 = Index Array(array=w254, index=w252) -> (element=w250:refnum<vi>)
  }
  n126 = for {
    tunnel: w11 -> [w269] mode=indexing
    tunnel: w10 -> [w266] mode=indexing
    tunnel: "Diagram" -> [w265]
    tunnel: [w264] -> w7 mode=indexing
    tunnel: w9 -> [w263]
    n127 = property class="Term"(reference=w269) -> ("Wire.Terms[]"=w268:refnum<vi>[], "IsSource"=w267:bool)  [unwired: 1 in, 2 out]
    n128 = case shown="False" w267 {
      tunnel: w268 -> [w279 _]
      tunnel: w266 -> [w273 w302]
      tunnel: w265 -> [w272 _]
      tunnel: [w271 w302] -> w264
      tunnel: w263 -> [w270 _]
      frame False {
        # "1st term is always source"
        n129 = Index Array(array=w279) -> (element=w278:refnum<vi>)  [unwired: 1 in]
        n130 = property class="Term"(reference=w278) -> ("Data Type"=w277:variant)  [unwired: 1 in, 2 out]
        n131 = call <vilib>:"exnSharedSub read variant type as a string.vi"("Variant"=w277) -> ("type as string"=w275:string)  [unwired: 14 in]
        n132 = Search 1D Array(1D array=string[] ["Waveform", "1D Array Waveform"], element=w275) -> (index of element=w274:i32)  [unwired: 1 in]
        n133 = case shown="Default" w274 {
          selector: w274 -> [_ w301]
          tunnel: w273 -> [w281 w300]
          tunnel: w272 -> [_ w295]
          tunnel: [w281 w283] -> w271
          tunnel: [w280 w288] -> _
          tunnel: w270 -> [w280 w286]
          frame -1 {
            # "Do not insert the \"To DDT\" if the input is not Waveform or a 1D Array of Waveforms."
          }
          frame Default {
            w293 = refnum<vi> refnum  # SubVI
            # "4"
            n134 = property class="Term"(reference=w300, error in=w286) -> (reference out=w291:refnum<vi>, error out=w287:errorcluster, "Position"=w299:T17)
            n135 = Index Array(array=path[] [path "<vilib>/express/express signal manip/ConverttoDDTBlocks.llb/Waveform to DDT.vi", path "<vilib>/express/express signal manip/ConverttoDDTBlocks.llb/1D Waveform to DDT.vi"], index=w301) -> (element=w285:path)
            n136 = Subtract(x=w299, y=T17 {"Left"=40, "Top"=0}) -> (x-y=w297:T17)
            n137 = New VI Object(vi object class=w293, owner refnum=w295, position/next to=w297, 6:w285, 8:w287) -> (object refnum=w294:refnum<vi>, 0:w290:errorcluster)  [unwired: 3 in]
            n138 = property class="SubVI"(reference=w294, error in=w290) -> (error out=w289:errorcluster, "Terms[]"=w292:refnum<vi>[])  [unwired: 1 out]
            n139 = Index Array(array=w292, index #1=2 ("index")) -> (element #1=w283:refnum<vi>, element #3=w282:refnum<vi>)  [unwired: 2 in, 1 out]
            n140 = invoke class="Term" method="Connect Wire"(reference=w282, error in=w289, "Wire Source"=w291) -> (error out=w288:errorcluster)  [unwired: 4 in, 6 out]
          }
        }
      }
      frame True {
        # "We don't care about output terminals."
      }
    }
  }
  n141 = for {
    tunnel: w84 -> [w304] mode=indexing
    tunnel: w7 -> [w305] mode=indexing
    shift-right: [w303] -> w39
    shift-left: w9 -> [w303]
    # "XNode term ref"
    # "subVI term ref"
    n142 = property class="Term"(reference=w304) -> ("Wire"=w307:refnum<vi>)  [unwired: 1 in, 2 out]
    n143 = Not A Number/Path/Refnum?(number/path/refnum=w307) -> (NaN/Path/Refnum?=w306:bool)
    n144 = case shown="False" w306 {
      tunnel: w304 -> [w309 _]
      tunnel: w305 -> [w308 _]
      frame False {
        n145 = invoke class="Term" method="Connect Wire"(reference=w308, "Wire Source"=w309) -> ()  [unwired: 5 in, 7 out]
      }
      frame True {
      }
    }
  }
  n146 = invoke class="SubVI" method="Delete"(reference=w91, error in=w39) -> (error out=w188:errorcluster)  [unwired: 1 in, 2 out]
  n147 = Unbundle By Name(w188) -> ("status"=w192:bool)
  n148 = Not(x=w192) -> (.not. x?=→"Replace?":bool)
